vi "Configure Websockets Connection.vi"(4 "Read Mode (Immediate)":T1(ring)=enum."Immediate", 5 "Connection.Websockets":refnum<class "Connection.WS.lvclass">, 6 "timeout (5000ms)":i32=5000, 7 "path (/)":string="/", 8 "error in (no error)":errorcluster, 9 "subProtocols":string[](array[string]), 10 "remote port (80)":u16=80, 11 "address (localhost)":string="localhost") -> (0 "error out":errorcluster, 3 "Connection.Websockets":refnum<class "Connection.WS.lvclass">)   [LabVIEW 2013, in "Connection.WS_GOSPL.lvlib" / "Connection.WS.lvclass"]
uses:
  Connection.WS.lvclass
  Connection.TCP/Connection.TCP.lvclass/Connection.TCP.ctl
  Connection.WS.lvclass/Connection.WS.ctl
  Connection/Connection.lvclass/Connection.ctl
  Connection/Connection.lvclass
  Connection.TCP/Connection.TCP.lvclass
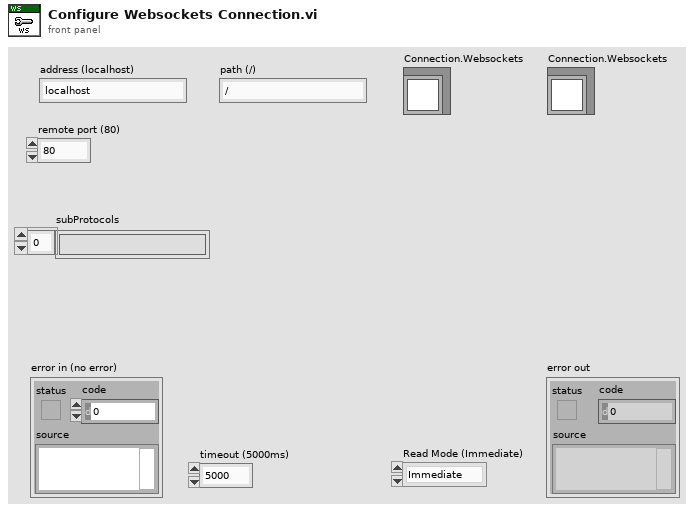
[diagram p1: front panel]
types:
  T1 = enum16{"Standard", "Buffered", "CRLF", "Immediate"}
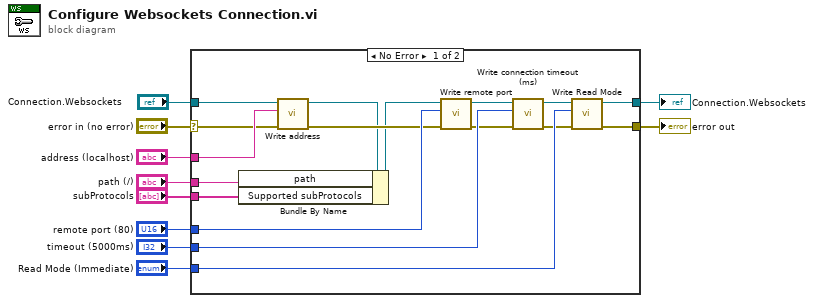
[diagram p0: block diagram]
diagram:
  n1 = case shown="No Error" "error in (no error)" {
    selector: "error in (no error)" -> [w15 w29]
    tunnel: [w19 w29] -> w9
    tunnel: [w21 w28] -> w5
    tunnel: "address (localhost)" -> [w24 _]
    tunnel: "remote port (80)" -> [w26 _]
    tunnel: "timeout (5000ms)" -> [w27 _]
    tunnel: "Read Mode (Immediate)" -> [w20 _]
    tunnel: "Connection.Websockets" -> [w25 w28]
    tunnel: "path (/)" -> [w14 _]
    tunnel: "subProtocols" -> [w11 _]
    frame No Error {
      n2 = call "Write address.vi"("error in (no error)"=w15, "address"=w24, "Connection.TCP"=w25) -> ("error out"=w16:errorcluster, "Connection.TCP"=w13:refnum<class "Connection.WS.lvclass">)  [unwired: 7 in]
      n3 = Bundle By Name(cluster=w13, "path"=w14, "Supported subProtocols"=w11) -> (w12:refnum<class "Connection.WS.lvclass">)
      n4 = call "Write remote port.vi"("error in (no error)"=w16, "remote port (80)"=w26, "Connection.TCP"=w12) -> ("error out"=w17:errorcluster, "Connection.TCP"=w23:refnum<class "Connection.WS.lvclass">)  [unwired: 7 in]
      n5 = call "Write connection timeout (ms).vi"("error in (no error)"=w17, "connection timeout (ms)"=w27, "Connection in"=w23) -> ("error out"=w18:errorcluster, "Connection out"=w22:refnum<class "Connection.WS.lvclass">)  [unwired: 7 in]
      n6 = call "Write Read Mode.vi"("error in (no error)"=w18, "Read Mode"=w20, "Connection.TCP"=w22) -> ("error out"=w19:errorcluster, "Connection.TCP"=w21:refnum<class "Connection.WS.lvclass">)  [unwired: 7 in]
    }
    frame Error {
    }
  }
  "error out" <- w9
  "Connection.Websockets" <- w5
